vi "AbortALL.vi"() -> ()   [LabVIEW 2012]
panel:
  out "Array":errorcluster[](array[cluster])
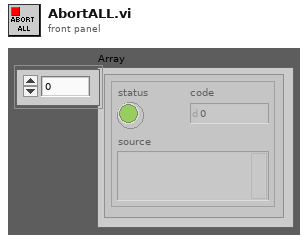
[diagram p1: front panel]
types:
  T1 = enum32{"Bad", "Idle", "Run top level", "Running"}
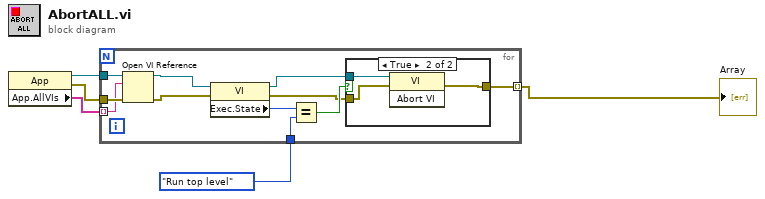
[diagram p0: block diagram]
diagram:
  n1 = property class="App"() -> (reference out=w4:refnum<vi>, error out=w5:errorcluster, "App.AllVIs"=w3:string[])  [unwired: 2 in]
  n2 = for {
    tunnel: w5 -> [w16]
    tunnel: w4 -> [w14]
    tunnel: w3 -> [w15] mode=indexing
    tunnel: [w13] -> w2 mode=indexing
    tunnel: T1."Run top level" ("Execution:State") -> [w10]
    n3 = Open VI Reference(application reference (local)=w14, vi path=w15, error in (no error)=w16) -> (vi reference=w11:refnum<vi>, error out=w12:errorcluster)  [unwired: 3 out]
    n4 = property class="VI"(reference=w11, error in=w12) -> (reference out=w8:refnum<vi>, error out=w6:errorcluster, "Exec.State"=w9:T1)
    n5 = Equal?(x=w9, y=w10) -> (x = y?=w7:bool)
    n6 = case shown="True" w7 {
      tunnel: [w17 w20] -> w13
      tunnel: w8 -> [_ w19]
      tunnel: w6 -> [w17 w18]
      frame False {
      }
      frame True {
        n7 = invoke class="VI" method="Abort VI"(reference=w19, error in=w18) -> (error out=w20:errorcluster)  [unwired: 1 in, 2 out]
      }
    }
  }
  "Array" <- w2
